vi "Estructuras Labview 2.vi"() -> ()   [LabVIEW 2022 SP3]
panel:
  in  "String 2":string
  out "Divisi":bool
  out "Multi":bool
  out "Operacion":string
  out "Resta":bool
  out "Suma":bool
  out "Resultado":dbl
  in  "Numeric 2":dbl
  in  "Numeric 1":dbl
  out "Iteraciones":i32
  in  "Stop Button":bool
  # "Se pide diseñar una claculadora de 2 operaciones"
  # "0 : Suma\n1 : Resta\n2 : Multiplicacion\n3 : Division"
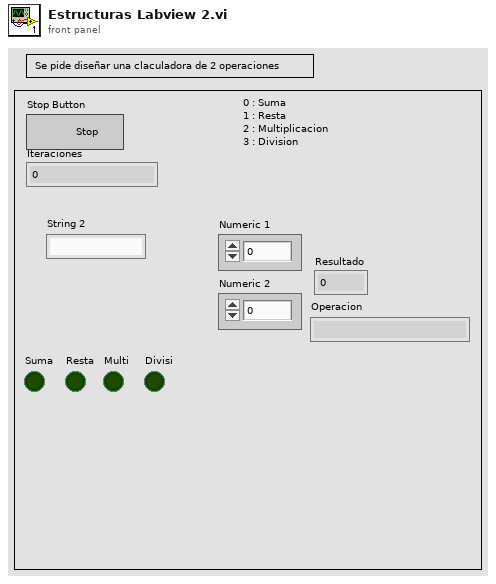
[diagram p1: front panel]
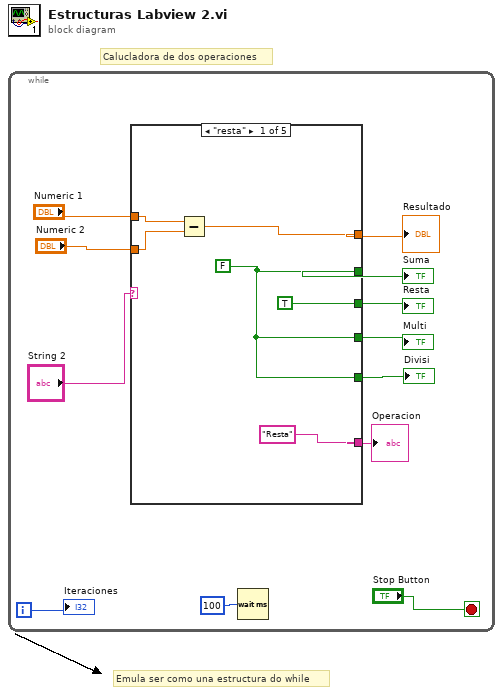
[diagram p0: block diagram]
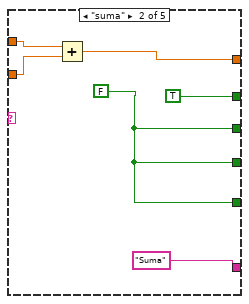
[diagram p2: hidden frame]
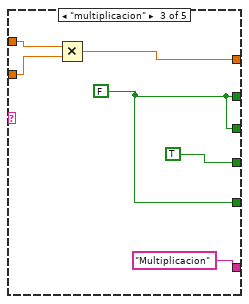
[diagram p3: hidden frame]
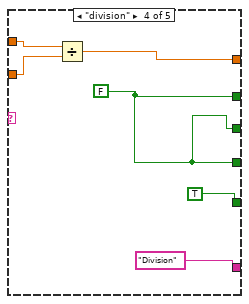
[diagram p4: hidden frame]
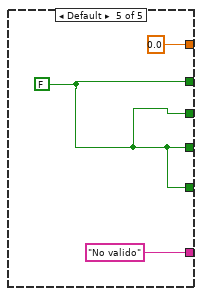
[diagram p5: hidden frame]
diagram:
  # "Emula ser como una estructura do while"
  # "Calucladora de dos operaciones"
  n1 = while {
    i -> [w11]
    stop <- "Stop Button" stop-if-true
    n2 = case shown="\"resta\"" "String 2" {
      tunnel: "Numeric 1" -> [w18 w24 w30 w36 _]
      tunnel: "Numeric 2" -> [w17 w23 w29 w35 _]
      tunnel: [w16 w22 w28 w34 0.0] -> w8
      tunnel: [w14 TRUE w26 w31 w37] -> w7
      tunnel: [TRUE w20 w26 w31 w37] -> w6
      tunnel: ["Resta" "Suma" "Multiplicacion" "Division" "No valido"] -> w2
      tunnel: [w14 w20 TRUE w31 w37] -> w4
      tunnel: [w14 w20 w26 TRUE w37] -> w3
      frame "resta" {
        w14 = FALSE
        n3 = Subtract(x=w18, y=w17) -> (x-y=w16:dbl)
      }
      frame "suma" {
        w20 = FALSE
        n4 = Add(x=w24, y=w23) -> (x+y=w22:dbl)
      }
      frame "multiplicacion" {
        w26 = FALSE
        n5 = Multiply(x=w30, y=w29) -> (x*y=w28:dbl)
      }
      frame "division" {
        w31 = FALSE
        n6 = Divide(x=w36, y=w35) -> (x/y=w34:dbl)
      }
      frame Default {
        w37 = FALSE
      }
    }
    "Resultado" <- w8
    "Suma" <- w7
    "Resta" <- w6
    "Operacion" <- w2
    "Multi" <- w4
    "Divisi" <- w3
    n7 = Wait (ms)(milliseconds to wait=u32 100) -> ()  [unwired: 1 out]
    "Iteraciones" <- w11
  }
